vi "ECT Calculation.vi"(0 "Option Selection":T2, 5 "ECT Parameters":T1, 11 "Error In":errorcluster) -> (4 "Expected ECT":T3, 15 "Error Out":errorcluster)   [LabVIEW 2016, in "2015 VA Washer.lvlib"]
uses:
  Projects/2015 VA Washer.lvlib
  Controls/ECT.ctl
  Controls/Options.ctl
  Controls/ECT Parameters.ctl
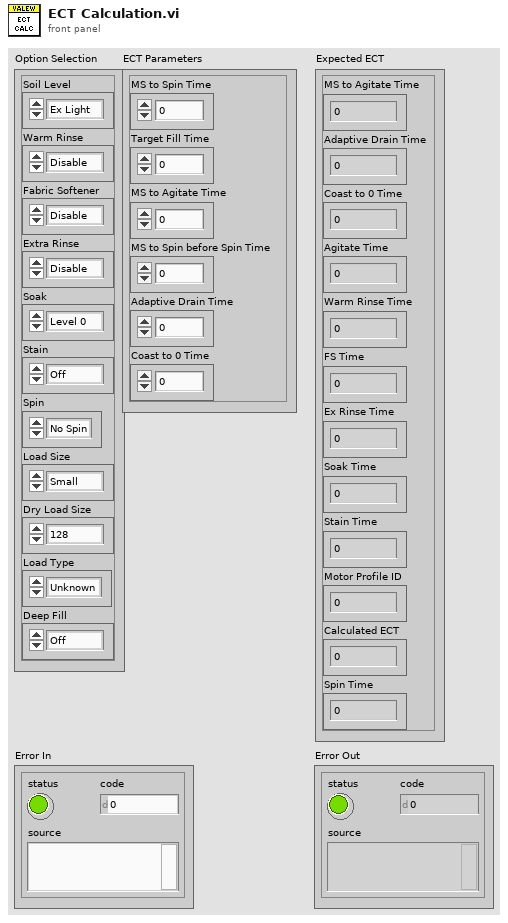
[diagram p1: front panel]
types:
  T1 = typedef "2015 VA Washer.lvlib/ECT Parameters.ctl" = cluster{"MS to Spin Time":u16, "Target Fill Time":u16, "MS to Agitate Time":u16, "MS to Spin before Spin Time ":u16, "Adaptive Drain Time":u16, "Coast to 0 Time":u16}
  T2 = typedef "2015 VA Washer.lvlib/Options.ctl" = cluster{"Soil Level":enum8{"Ex Light", "Light", "Normal", "Heavy", "Ex Heavy"}, "Warm Rinse":enum8{"Disable", "Enable"}, "Fabric Softener":enum16{"Disable", "Enable"}, "Extra Rinse":enum8{"Disable", "Enable"}, "Soak":enum8{"Level 0", "Level 1", "Level 2", "Level 3", "Level 4"}, "Stain":enum8{"Off", "Tomato", "Wine", "Blood", "Grass", "Dirt"}, "Spin":enum16{"No Spin", "Normal Spin", "More Spin", "Max Spin"}, "Load Size":enum8{"Small", "Medium", "Large", "Super", "Precise Fill", "Super Plus"}, "Dry Load Size":enum16{"128", "256", "384", "5AA", "6A4", "834", "65535"}, "Load Type":enum8{"Unknown", "Cotton", "Synthetic", "Mixed", "Wet", "Low Flow", "Small", "Medium", "Large", "Super", "Super Plus", "Max"}, "Deep Fill":enum8{"Off", "Incremental Fill", "Max Fill"}}
  T3 = typedef "2015 VA Washer.lvlib/ECT.ctl" = cluster{"MS to Agitate Time":u16, "Adaptive Drain Time":u16, "Coast to 0 Time":u16, "Agitate Time":u16, "Warm Rinse Time":u16, "FS Time":u16, "Ex Rinse Time":u16, "Soak Time":u16, "Stain Time":u16, "Motor Profile ID":u16, "Calculated ECT":u16, "Spin Time":u16}
  T4 = enum8{"Small", "Medium", "Large", "Super", "Precise Fill", "Super Plus"}
  T5 = enum8{"Level 0", "Level 1", "Level 2", "Level 3", "Level 4"}
  T6 = enum8{"Off", "Tomato", "Wine", "Blood", "Grass", "Dirt"}
  T7 = enum16{"No Spin", "Normal Spin", "More Spin", "Max Spin"}
  T8 = enum16{"128", "256", "384", "5AA", "6A4", "834", "65535"}
  T9 = enum8{"Unknown", "Cotton", "Synthetic", "Mixed", "Wet", "Low Flow", "Small", "Medium", "Large", "Super", "Super Plus", "Max"}
  T10 = enum8{"Ex Light", "Light", "Normal", "Heavy", "Ex Heavy"}
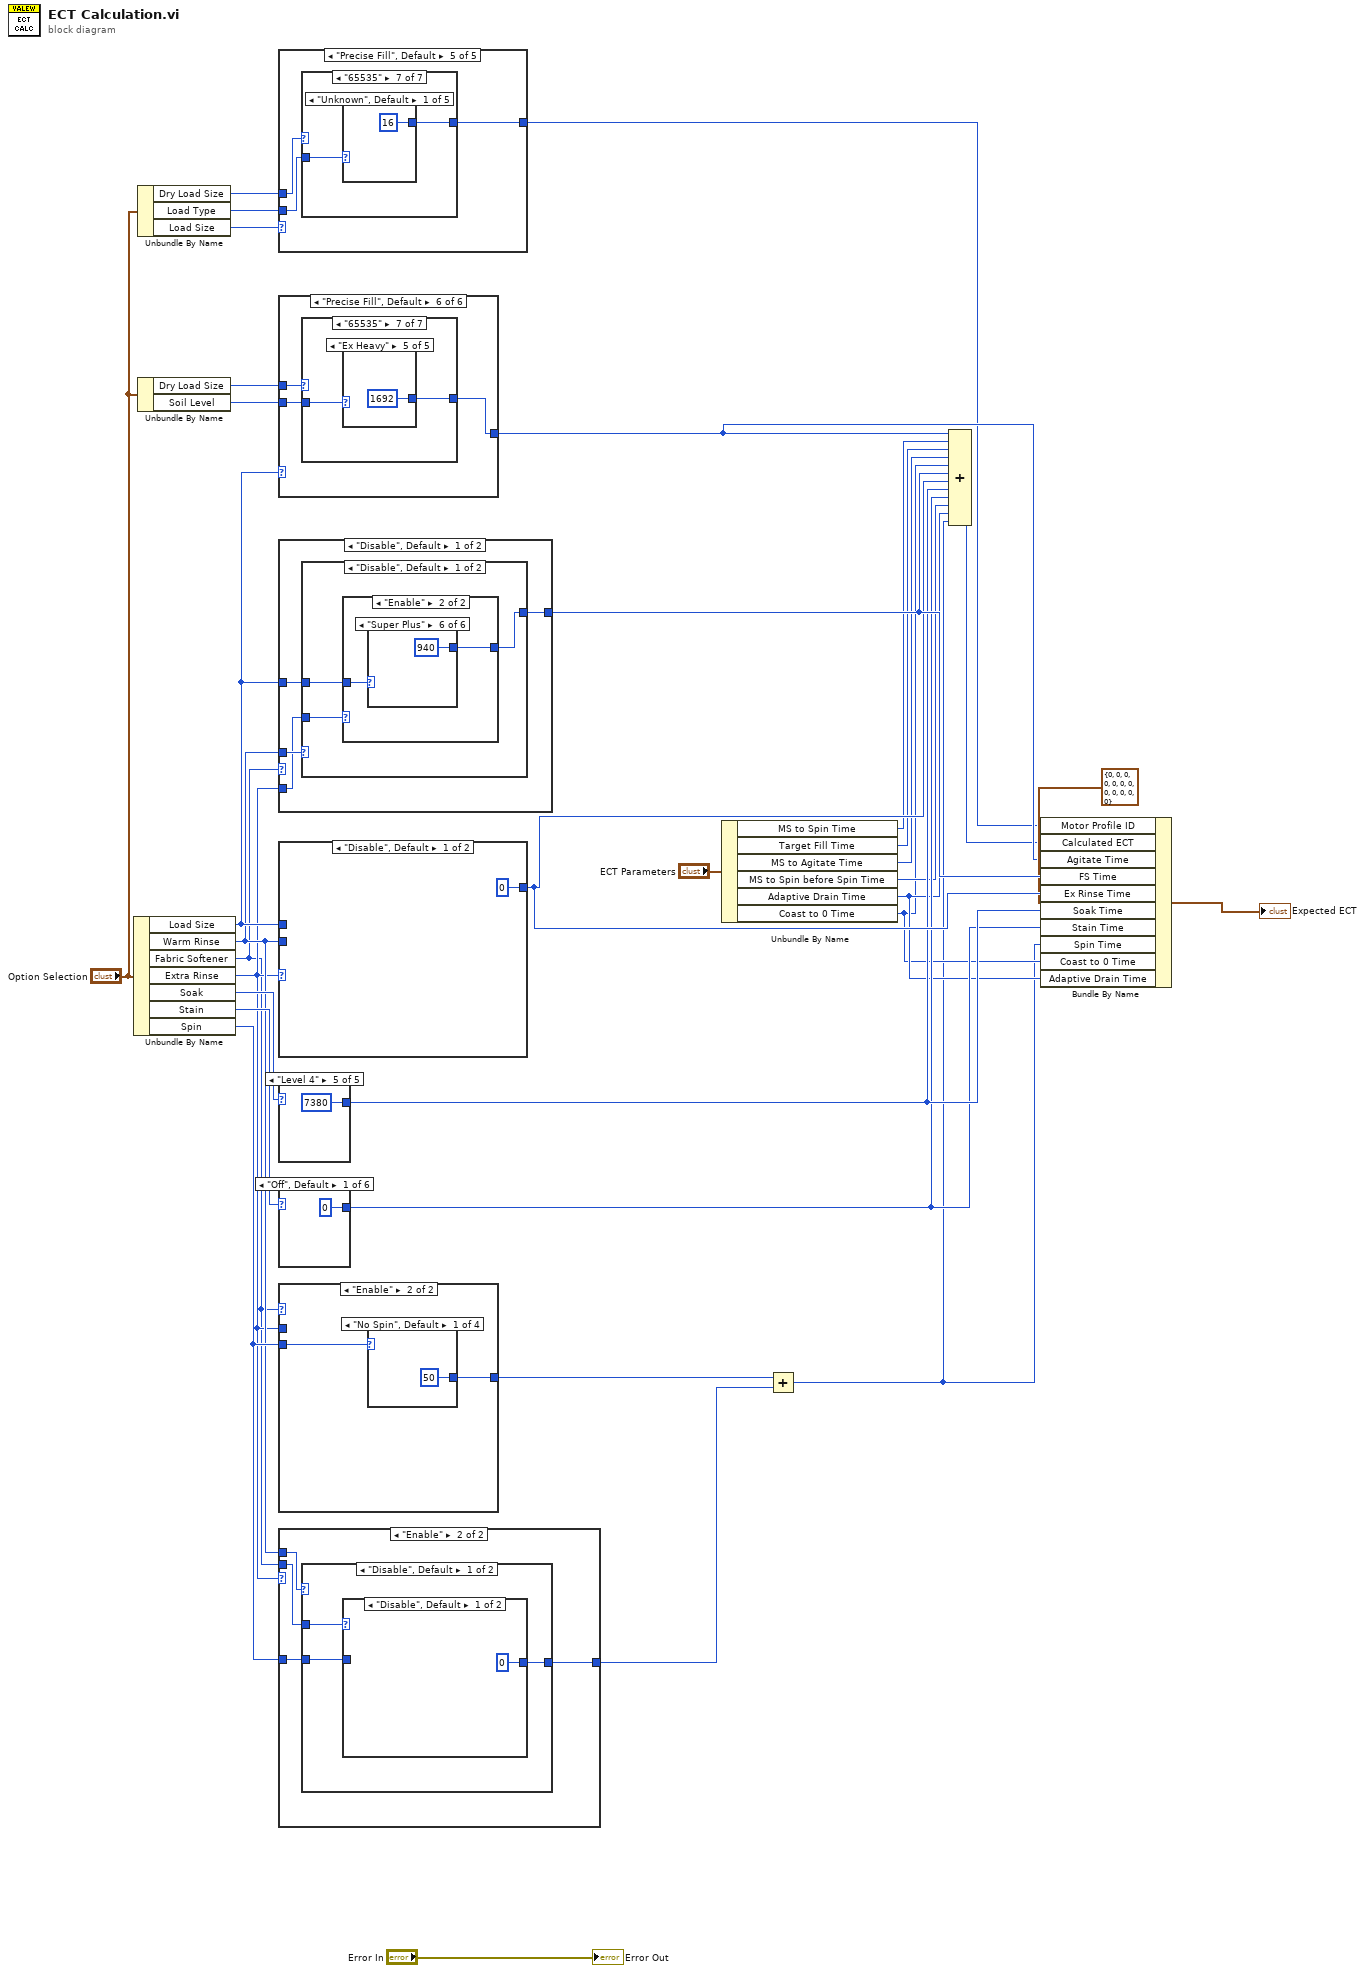
[diagram p0: block diagram]
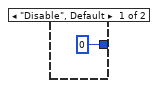
[diagram p2: hidden frame]
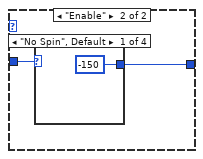
[diagram p3: hidden frame]
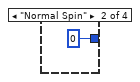
[diagram p4: hidden frame]
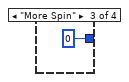
[diagram p5: hidden frame]
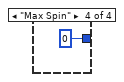
[diagram p6: hidden frame]
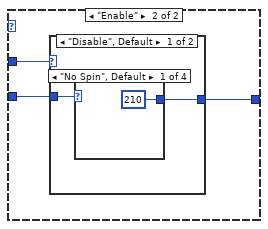
[diagram p7: hidden frame]
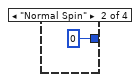
[diagram p8: hidden frame]
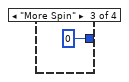
[diagram p9: hidden frame]
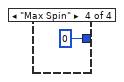
[diagram p10: hidden frame]
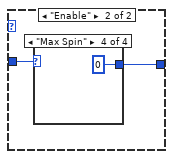
[diagram p11: hidden frame]
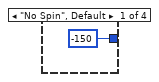
[diagram p12: hidden frame]
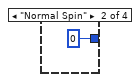
[diagram p13: hidden frame]
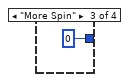
[diagram p14: hidden frame]
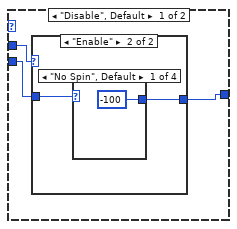
[diagram p15: hidden frame]
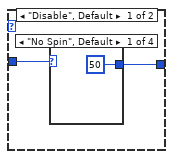
[diagram p16: hidden frame]
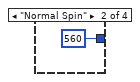
[diagram p17: hidden frame]
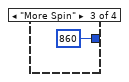
[diagram p18: hidden frame]
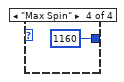
[diagram p19: hidden frame]
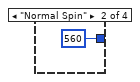
[diagram p20: hidden frame]
diagram:
  n1 = Unbundle By Name("Option Selection") -> ("Load Size"=w8:T4, "Warm Rinse"=w6:enum8{"Disable", "Enable"}, "Fabric Softener"=w4:enum16{"Disable", "Enable"}, "Extra Rinse"=w5:enum8{"Disable", "Enable"}, "Soak"=w32:T5, "Stain"=w33:T6, "Spin"=w7:T7)
  n2 = Unbundle By Name("Option Selection") -> ("Dry Load Size"=w29:T8, "Load Type"=w28:T9, "Load Size"=w10:T4)
  n3 = Unbundle By Name("Option Selection") -> ("Dry Load Size"=w30:T8, "Soil Level"=w31:T10)
  n4 = case shown="\"Precise Fill\", Default" w10 {
    tunnel: [u16 16 u16 19 u16 21 u16 23 w40] -> w17
    tunnel: w29 -> [_ _ _ _ w39]
    tunnel: w28 -> [_ _ _ _ w38]
    frame "Small" {
    }
    frame "Medium" {
    }
    frame "Large" {
    }
    frame "Super" {
    }
    frame "Precise Fill", Default {
      n5 = case shown="\"65535\"" w39 {
        tunnel: [w41 w49 w56 w63 w70 _ w77] -> w40
        tunnel: w38 -> [w42 w48 w55 w62 w69 _ w76]
        frame "128", Default {
          n6 = case shown="\"Wet\"" w42 {
            tunnel: [u16 16 u16 18 u16 19 u16 20 u16 25] -> w41
            frame "Unknown", Default {
            }
            frame "Cotton" {
            }
            frame "Synthetic" {
            }
            frame "Mixed" {
            }
            frame "Wet" {
            }
          }
        }
        frame "256" {
          n7 = case shown="\"Wet\"" w48 {
            tunnel: [u16 16 u16 22 u16 23 u16 24 u16 25] -> w49
            frame "Unknown", Default {
            }
            frame "Cotton" {
            }
            frame "Synthetic" {
            }
            frame "Mixed" {
            }
            frame "Wet" {
            }
          }
        }
        frame "384" {
          n8 = case shown="\"Wet\"" w55 {
            tunnel: [u16 16 u16 25 u16 24 u16 23 u16 22] -> w56
            frame "Unknown", Default {
            }
            frame "Cotton" {
            }
            frame "Synthetic" {
            }
            frame "Mixed" {
            }
            frame "Wet" {
            }
          }
        }
        frame "5AA" {
          n9 = case shown="\"Wet\"" w62 {
            tunnel: [u16 16 u16 2 u16 16 u16 18 u16 19] -> w63
            frame "Unknown", Default {
            }
            frame "Cotton" {
            }
            frame "Synthetic" {
            }
            frame "Mixed" {
            }
            frame "Wet" {
            }
          }
        }
        frame "6A4" {
          n10 = case shown="\"Synthetic\"" w69 {
            tunnel: [u16 16 u16 16 u16 20 u16 2 u16 21] -> w70
            frame "Unknown", Default {
            }
            frame "Cotton" {
            }
            frame "Synthetic" {
            }
            frame "Mixed" {
            }
            frame "Wet" {
            }
          }
        }
        frame "834" {
        }
        frame "65535" {
          n11 = case shown="\"Unknown\", Default" w76 {
            tunnel: [u16 16 u16 2 u16 18 u16 21 u16 22] -> w77
            frame "Unknown", Default {
            }
            frame "Cotton" {
            }
            frame "Synthetic" {
            }
            frame "Mixed" {
            }
            frame "Wet" {
            }
          }
        }
      }
    }
  }
  n12 = case shown="\"Precise Fill\", Default" w8 {
    tunnel: w31 -> [w84 w91 w98 w105 w112 w119]
    tunnel: w30 -> [_ _ _ _ _ w120]
    tunnel: [w83 w90 w97 w104 w111 w118] -> w19
    frame "Small" {
      n13 = case shown="\"Light\", Default" w84 {
        tunnel: [u16 360 u16 480 u16 720 u16 1440 u16 1680] -> w83
        frame "Ex Light" {
        }
        frame "Light", Default {
        }
        frame "Normal" {
        }
        frame "Heavy" {
        }
        frame "Ex Heavy" {
        }
      }
    }
    frame "Medium" {
      n14 = case shown="\"Ex Heavy\"" w91 {
        tunnel: [u16 360 u16 480 u16 720 u16 1440 u16 1680] -> w90
        frame "Ex Light" {
        }
        frame "Light", Default {
        }
        frame "Normal" {
        }
        frame "Heavy" {
        }
        frame "Ex Heavy" {
        }
      }
    }
    frame "Large" {
      n15 = case shown="\"Ex Heavy\"" w98 {
        tunnel: [u16 480 u16 600 u16 840 u16 1560 u16 1800] -> w97
        frame "Ex Light" {
        }
        frame "Light", Default {
        }
        frame "Normal" {
        }
        frame "Heavy" {
        }
        frame "Ex Heavy" {
        }
      }
    }
    frame "Super" {
      n16 = case shown="\"Heavy\"" w105 {
        tunnel: [u16 600 u16 720 u16 960 u16 1680 u16 1800] -> w104
        frame "Ex Light" {
        }
        frame "Light", Default {
        }
        frame "Normal" {
        }
        frame "Heavy" {
        }
        frame "Ex Heavy" {
        }
      }
    }
    frame "Super Plus" {
      n17 = case shown="\"Ex Heavy\"" w112 {
        tunnel: [u16 660 u16 840 u16 1080 u16 1800 u16 1800] -> w111
        frame "Ex Light" {
        }
        frame "Light", Default {
        }
        frame "Normal" {
        }
        frame "Heavy" {
        }
        frame "Ex Heavy" {
        }
      }
    }
    frame "Precise Fill", Default {
      n18 = case shown="\"65535\"" w120 {
        tunnel: w119 -> [w122 w129 w136 w143 w150 w157 w163]
        tunnel: [w121 w128 w135 w142 w149 w156 w164] -> w118
        frame "128", Default {
          n19 = case shown="\"Ex Heavy\"" w122 {
            tunnel: [u16 360 u16 480 u16 720 u16 1440 u16 1680] -> w121
            frame "Ex Light" {
            }
            frame "Light", Default {
            }
            frame "Normal" {
            }
            frame "Heavy" {
            }
            frame "Ex Heavy" {
            }
          }
        }
        frame "256" {
          n20 = case shown="\"Ex Heavy\"" w129 {
            tunnel: [u16 360 u16 480 u16 720 u16 1440 u16 1680] -> w128
            frame "Ex Light" {
            }
            frame "Light", Default {
            }
            frame "Normal" {
            }
            frame "Heavy" {
            }
            frame "Ex Heavy" {
            }
          }
        }
        frame "384" {
          n21 = case shown="\"Ex Heavy\"" w136 {
            tunnel: [u16 360 u16 480 u16 720 u16 1440 u16 1680] -> w135
            frame "Ex Light" {
            }
            frame "Light", Default {
            }
            frame "Normal" {
            }
            frame "Heavy" {
            }
            frame "Ex Heavy" {
            }
          }
        }
        frame "5AA" {
          n22 = case shown="\"Ex Heavy\"" w143 {
            tunnel: [u16 480 u16 600 u16 840 u16 1560 u16 1800] -> w142
            frame "Ex Light" {
            }
            frame "Light", Default {
            }
            frame "Normal" {
            }
            frame "Heavy" {
            }
            frame "Ex Heavy" {
            }
          }
        }
        frame "6A4" {
          n23 = case shown="\"Heavy\"" w150 {
            tunnel: [u16 600 u16 720 u16 960 u16 1680 u16 1800] -> w149
            frame "Ex Light" {
            }
            frame "Light", Default {
            }
            frame "Normal" {
            }
            frame "Heavy" {
            }
            frame "Ex Heavy" {
            }
          }
        }
        frame "834" {
          n24 = case shown="\"Ex Heavy\"" w157 {
            tunnel: [u16 660 u16 840 u16 1080 u16 1800 u16 1800] -> w156
            frame "Ex Light" {
            }
            frame "Light", Default {
            }
            frame "Normal" {
            }
            frame "Heavy" {
            }
            frame "Ex Heavy" {
            }
          }
        }
        frame "65535" {
          n25 = case shown="\"Ex Heavy\"" w163 {
            tunnel: [u16 372 u16 492 u16 732 u16 1452 u16 1692] -> w164
            frame "Ex Light" {
            }
            frame "Light", Default {
            }
            frame "Normal" {
            }
            frame "Heavy" {
            }
            frame "Ex Heavy" {
            }
          }
        }
      }
    }
  }
  n26 = case shown="\"Disable\", Default" w4 {
    tunnel: [w171 w202] -> w26
    tunnel: w5 -> [w170 w204]
    tunnel: w8 -> [w172 w203]
    tunnel: w6 -> [w173 w201]
    frame "Disable", Default {
      n27 = case shown="\"Disable\", Default" w173 {
        tunnel: [w176 w194] -> w171
        tunnel: w172 -> [w175 w193]
        tunnel: w170 -> [w174 _]
        frame "Disable", Default {
          n28 = case shown="\"Enable\"" w174 {
            tunnel: [w177 w186] -> w176
            tunnel: w175 -> [w178 w185]
            frame "Disable", Default {
              n29 = case shown="\"Precise Fill\"" w178 {
                tunnel: [u16 360 u16 510 u16 630 u16 730 u16 510 u16 730] -> w177
                frame "Small", Default {
                }
                frame "Medium" {
                }
                frame "Large" {
                }
                frame "Super" {
                }
                frame "Precise Fill" {
                }
                frame "Super Plus" {
                }
              }
            }
            frame "Enable" {
              n30 = case shown="\"Super Plus\"" w185 {
                tunnel: [u16 570 u16 720 u16 840 u16 940 u16 720 u16 940] -> w186
                frame "Small", Default {
                }
                frame "Medium" {
                }
                frame "Large" {
                }
                frame "Super" {
                }
                frame "Precise Fill" {
                }
                frame "Super Plus" {
                }
              }
            }
          }
        }
        frame "Enable" {
          n31 = case shown="\"Super Plus\"" w193 {
            tunnel: [u16 395 u16 510 u16 600 u16 675 u16 510 u16 675] -> w194
            frame "Small", Default {
            }
            frame "Medium" {
            }
            frame "Large" {
            }
            frame "Super" {
            }
            frame "Precise Fill" {
            }
            frame "Super Plus" {
            }
          }
        }
      }
    }
    frame "Enable" {
      n32 = case shown="\"Disable\", Default" w204 {
        tunnel: w203 -> [w207 w225]
        tunnel: [w205 w224] -> w202
        tunnel: w201 -> [w206 _]
        frame "Disable", Default {
          n33 = case shown="\"Enable\"" w206 {
            tunnel: [w209 w217] -> w205
            tunnel: w207 -> [w208 w216]
            frame "Disable", Default {
              n34 = case shown="\"Super Plus\"" w208 {
                tunnel: [u16 1028 u16 1178 u16 1298 u16 1398 u16 1178 u16 1398] -> w209
                frame "Small", Default {
                }
                frame "Medium" {
                }
                frame "Large" {
                }
                frame "Super" {
                }
                frame "Precise Fill" {
                }
                frame "Super Plus" {
                }
              }
            }
            frame "Enable" {
              n35 = case shown="\"Super Plus\"" w216 {
                tunnel: [u16 983 u16 1098 u16 1188 u16 1263 u16 1098 u16 1263] -> w217
                frame "Small", Default {
                }
                frame "Medium" {
                }
                frame "Large" {
                }
                frame "Super" {
                }
                frame "Precise Fill" {
                }
                frame "Super Plus" {
                }
              }
            }
          }
        }
        frame "Enable" {
          n36 = case shown="\"Super Plus\"" w225 {
            tunnel: [u16 1195 u16 1345 u16 1465 u16 1565 u16 1345 u16 1565] -> w224
            frame "Small", Default {
            }
            frame "Medium" {
            }
            frame "Large" {
            }
            frame "Super" {
            }
            frame "Precise Fill" {
            }
            frame "Super Plus" {
            }
          }
        }
      }
    }
  }
  n37 = case shown="\"Disable\", Default" w5 {
    tunnel: [u16 0 w233] -> w25
    tunnel: w6 -> [_ w235]
    tunnel: w8 -> [_ w234]
    frame "Disable", Default {
    }
    frame "Enable" {
      n38 = case shown="\"Disable\", Default" w235 {
        tunnel: w234 -> [w237 w245]
        tunnel: [w236 w244] -> w233
        frame "Disable", Default {
          n39 = case shown="\"Super Plus\"" w237 {
            tunnel: [u16 570 u16 720 u16 840 u16 940 u16 720 u16 940] -> w236
            frame "Small", Default {
            }
            frame "Medium" {
            }
            frame "Large" {
            }
            frame "Super" {
            }
            frame "Precise Fill" {
            }
            frame "Super Plus" {
            }
          }
        }
        frame "Enable" {
          n40 = case shown="\"Super Plus\"" w245 {
            tunnel: [u16 525 u16 640 u16 730 u16 805 u16 640 u16 805] -> w244
            frame "Small", Default {
            }
            frame "Medium" {
            }
            frame "Large" {
            }
            frame "Super" {
            }
            frame "Precise Fill" {
            }
            frame "Super Plus" {
            }
          }
        }
      }
    }
  }
  n41 = case shown="\"Level 4\"" w32 {
    tunnel: [u16 0 u16 1080 u16 1980 u16 3780 u16 7380] -> w24
    frame "Level 0", Default {
    }
    frame "Level 1" {
    }
    frame "Level 2" {
    }
    frame "Level 3" {
    }
    frame "Level 4" {
    }
  }
  n42 = case shown="\"Off\", Default" w33 {
    tunnel: [u16 0 u16 1200 u16 1200 u16 1200 u16 1200 u16 1200] -> w23
    frame "Off", Default {
    }
    frame "Tomato" {
    }
    frame "Wine" {
    }
    frame "Blood" {
    }
    frame "Grass" {
    }
    frame "Dirt" {
    }
  }
  n43 = case shown="\"Enable\"" w4 {
    tunnel: [w264 w279] -> w2
    tunnel: w7 -> [w263 w278]
    tunnel: w5 -> [w265 _]
    frame "Disable", Default {
      n44 = case shown="\"Enable\"" w265 {
        tunnel: [w266 w273] -> w264
        tunnel: w263 -> [w267 w272]
        frame "Disable", Default {
          n45 = case shown="\"No Spin\", Default" w267 {
            tunnel: [u16 50 u16 560 u16 860 u16 1160] -> w266
            frame "No Spin", Default {
            }
            frame "Normal Spin" {
            }
            frame "More Spin" {
            }
            frame "Max Spin" {
            }
          }
        }
        frame "Enable" {
          n46 = case shown="\"No Spin\", Default" w272 {
            tunnel: [i16 -100 u16 560 u16 860 u16 1160] -> w273
            frame "No Spin", Default {
            }
            frame "Normal Spin" {
            }
            frame "More Spin" {
            }
            frame "Max Spin" {
            }
          }
        }
      }
    }
    frame "Enable" {
      n47 = case shown="\"No Spin\", Default" w278 {
        tunnel: [u16 50 u16 560 u16 860 u16 1160] -> w279
        frame "No Spin", Default {
        }
        frame "Normal Spin" {
        }
        frame "More Spin" {
        }
        frame "Max Spin" {
        }
      }
    }
  }
  n48 = case shown="\"Enable\"" w5 {
    tunnel: w7 -> [_ w288]
    tunnel: w6 -> [_ w285]
    tunnel: w4 -> [_ w286]
    tunnel: [u16 0 w287] -> w1
    frame "Disable", Default {
    }
    frame "Enable" {
      n49 = case shown="\"Disable\", Default" w285 {
        tunnel: w288 -> [w290 w301]
        tunnel: [w289 w300] -> w287
        tunnel: w286 -> [w291 w299]
        frame "Disable", Default {
          n50 = case shown="\"Disable\", Default" w291 {
            tunnel: w290 -> [_ w294]
            tunnel: [u16 0 w293] -> w289
            frame "Disable", Default {
            }
            frame "Enable" {
              n51 = case shown="\"No Spin\", Default" w294 {
                tunnel: [i16 -150 u16 0 u16 0 u16 0] -> w293
                frame "No Spin", Default {
                }
                frame "Normal Spin" {
                }
                frame "More Spin" {
                }
                frame "Max Spin" {
                }
              }
            }
          }
        }
        frame "Enable" {
          n52 = case shown="\"Disable\", Default" w299 {
            tunnel: w301 -> [w302 w309]
            tunnel: [w303 w308] -> w300
            frame "Disable", Default {
              n53 = case shown="\"No Spin\", Default" w302 {
                tunnel: [u16 210 u16 0 u16 0 u16 0] -> w303
                frame "No Spin", Default {
                }
                frame "Normal Spin" {
                }
                frame "More Spin" {
                }
                frame "Max Spin" {
                }
              }
            }
            frame "Enable" {
              n54 = case shown="\"Max Spin\"" w309 {
                tunnel: [i16 -150 u16 0 u16 0 u16 0] -> w308
                frame "No Spin", Default {
                }
                frame "Normal Spin" {
                }
                frame "More Spin" {
                }
                frame "Max Spin" {
                }
              }
            }
          }
        }
      }
    }
  }
  n55 = Unbundle By Name("ECT Parameters") -> ("MS to Spin Time"=w15:u16, "Target Fill Time"=w14:u16, "MS to Agitate Time"=w13:u16, "MS to Spin before Spin Time"=w12:u16, "Adaptive Drain Time"=w11:u16, "Coast to 0 Time"=w9:u16)
  n56 = Add(x=w2, y=w1) -> (x+y=w3:u16)
  n57 = Compound Arithmetic op=ADD(w19, w15, w14, w13, w9, w26, w25, w24, w23, w12, w11, w3) -> (w18:u16)
  n58 = Bundle By Name(cluster=T3 {"MS to Agitate Time"=0, "Adaptive Drain Time"=0, "Coast to 0 Time"=0, "Agitate Time"=0, "Warm Rinse Time"=0, "FS Time"=0, "Ex Rinse Time"=0, "Soak Time"=0, "Stain Time"=0, "Motor Profile ID"=0, "Calculated ECT"=0, "Spin Time"=0} ("Estimated Cycle Time 2"), "Motor Profile ID"=w17, "Calculated ECT"=w18, "Agitate Time"=w19, "FS Time"=w26, "Ex Rinse Time"=w25, "Soak Time"=w24, "Stain Time"=w23, "Spin Time"=w3, "Coast to 0 Time"=w9, "Adaptive Drain Time"=w11) -> (→"Expected ECT":T3)
  "Error Out" <- "Error In"
